vi "Histogram i gsto prawdopodobiestwa.vi"(9 "Liczba probek":i32, 10 "Wyjscie":dbl[](array[numeric]), 11 "co ile":dbl) -> (1 "Dystrybuanta":cluster{dbl[], dbl[]}(graph), 2 "Gêstoœæ prawdopodobieñstwa":cluster{dbl[], dbl[]}(graph), 3 "Histogram":cluster{dbl[], i32[]}(graph))   [LabVIEW 2019]
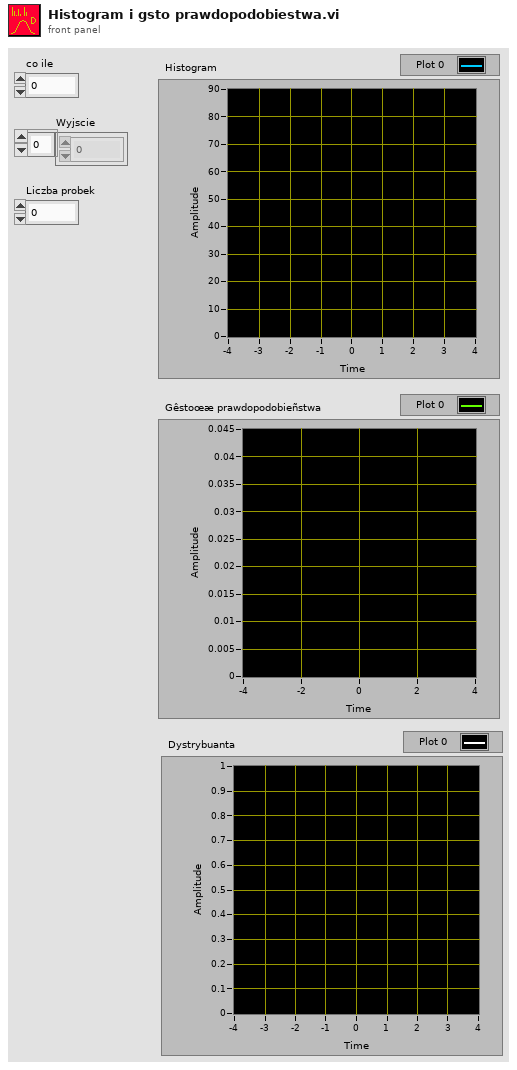
[diagram p1: front panel]
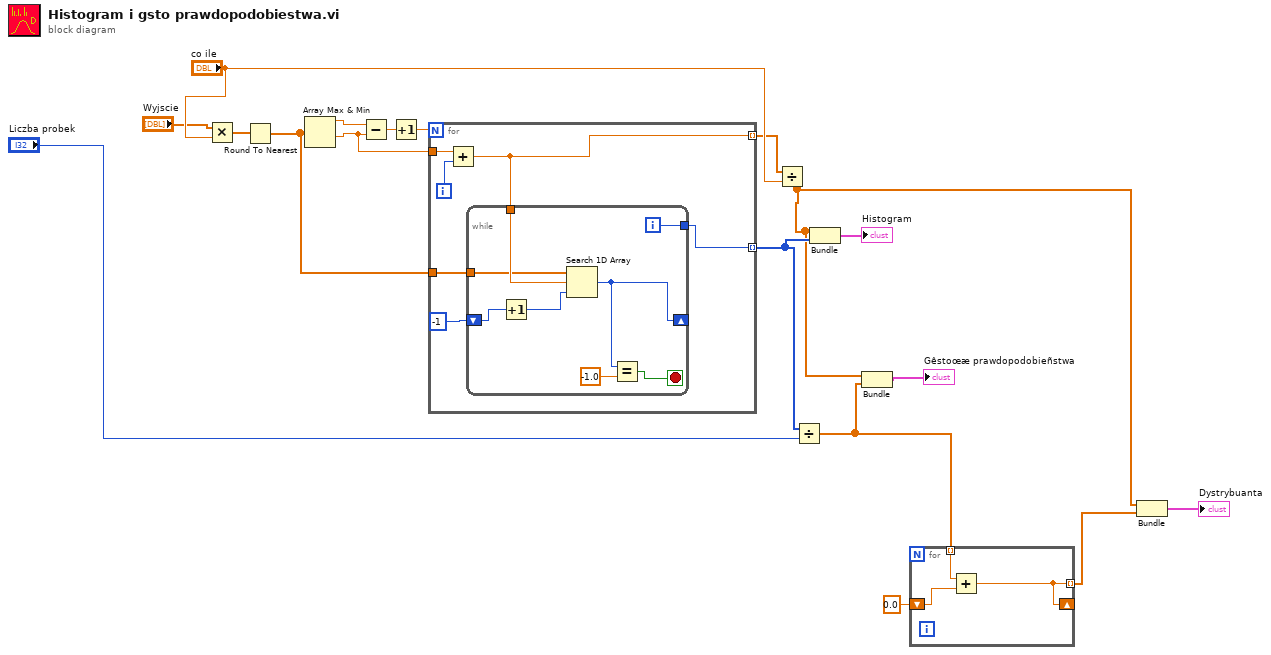
[diagram p0: block diagram]
diagram:
  n1 = Multiply(x="Wyjscie", y="co ile") -> (x*y=w14:dbl[])
  n2 = Round To Nearest(number=w14) -> (nearest integer value=w15:dbl[])
  n3 = Array Max & Min(array=w15) -> (max value=w7:dbl, min value=w8:dbl)  [unwired: 2 out]
  n4 = Subtract(x=w7, y=w8) -> (x-y=w10:dbl)
  n5 = Increment(x=w10) -> (x+1=w11:dbl)
  n6 = for {
    N: w11 -> [_]
    tunnel: w8 -> [w24]
    tunnel: [w21] -> w13 mode=indexing
    tunnel: w15 -> [w22]
    tunnel: [w19] -> w5 mode=indexing
    i -> [w23]
    n7 = Add(x=w24, y=w23) -> (x+y=w21:dbl)
    n8 = while {
      tunnel: w22 -> [w27]
      tunnel: w21 -> [w30]
      shift-right: [w29] -> _
      shift-left: -1 ("start index (0)") -> [w26]
      tunnel: [w28] -> w19
      i -> [w28]
      stop <- w31 stop-if-true
      n9 = Increment(x=w26) -> (x+1=w25:i32)
      n10 = Search 1D Array(1D array=w27, element=w30, start index (0)=w25) -> (index of element=w29:i32)
      n11 = Equal?(x=w29, y=-1.0) -> (x = y?=w31:bool)
    }
  }
  n12 = Divide(x=w13, y="co ile") -> (x/y=w2:dbl[])
  n13 = Divide(x=w5, y="Liczba probek") -> (x/y=w1:dbl[])
  n14 = Bundle(w2, w5) -> (→"Histogram":cluster{dbl[], i32[]})  [unwired: 1 in]
  n15 = Bundle(w2, w1) -> (→"Gêstoœæ prawdopodobieñstwa":cluster{dbl[], dbl[]})  [unwired: 1 in]
  n16 = for {
    shift-right: [w34] -> _
    shift-left: 0.0 -> [w35]
    tunnel: [w34] -> w4 mode=indexing
    tunnel: w1 -> [w33] mode=indexing
    n17 = Add(x=w33, y=w35) -> (x+y=w34:dbl)
  }
  n18 = Bundle(w2, w4) -> (→"Dystrybuanta":cluster{dbl[], dbl[]})  [unwired: 1 in]
